vi "Result Database Logging Engine.vi"(11 "Sequence Context":T1) -> (0 "error out":errorcluster)   [LabVIEW 2023, in "HardwareAbstractionLayer_LVOOP.lvlib" / "Report.lvclass"]
uses:
  Report.lvclass
  Report.lvclass/Report.ctl
  Database/Database.lvclass
  Database/SQL Public VI/Control/DB Options.ctl
  Control/Q Data.ctl
  Control/UUT Test Info.ctl
  Control/FE FRAME LOG.ctl
  Control/LIMIT TABLE.ctl
  Control/ERROR LOG.ctl
  Teststand/Teststand.lvclass
  Control/FF FRAME LOG.ctl
  Control/FA FRAME LOG.ctl
  Control/ERROR LOG APPEND.ctl
  Control/TEST RESULT LOG.ctl
  Control/TEST RESULT LOG APPEND.ctl
  Control/SYSTEM LOG.ctl
  Control/Temperature LOG.ctl
  Control/POWER STATUS.ctl
  Control/CYCLE_DURATION_LOG.ctl
  Control/FE FF DECODER.ctl
  <vilib>/addons/TestStand/_TSUtility.llb/TestStand - Get Property Value (Boolean).vi
  Control/Queue FGV.ctl
  <vilib>/addons/TestStand/_TSLegacy.llb/LabVIEW Test - Sequence Context.ctl
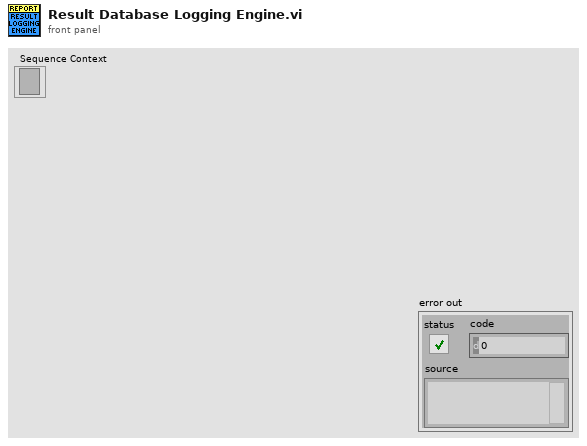
[diagram p1: front panel]
types:
  T1 = typedef "LabVIEW Test - Sequence Context.ctl" = refnum<k7>
  T2 = typedef "HardwareAbstractionLayer_LVOOP.lvlib/Report.lvclass/Queue FGV.ctl" = enum16{"Init", "Set", "Get"}
  T3 = typedef "HardwareAbstractionLayer_LVOOP.lvlib/Database.lvclass/DB Options.ctl" = enum16{"Init", "Select Data", "Insert Data", "Update Data", "Delete Data", "Execute Query", "Create Schema", "Create Table", "List Tables", "List Columns", "Close"}
  T4 = typedef "HardwareAbstractionLayer_LVOOP.lvlib/Report.lvclass/Q Data.ctl" = cluster{"Table Name":string, "Data":variant, "Action":enum16{"Insert", "Update"}, "Schema":string, "Socket No":u16}
  T5 = typedef "TestStand - Status Monitor.ctl" = cluster{"Sequence Context":refnum<k7>, "Execution":refnum<k7>, "Termination Monitor":refnum<k7>}
  T6 = typedef "HardwareAbstractionLayer_LVOOP.lvlib/Report.lvclass/UUT Test Info.ctl" = cluster{"ID":string, "STATION_ID":string, "TEST_SOCKET_INDEX":string, "UUT_SERIAL_NUMBER":string, "TSW_VER":string, "VAL_SW_VER":string, "PROJECT_NAME":string, "PRODUCT_NAME":string, "PRODUCT_VARIANT":string, "TEST_NAME":string, "TEST_PHASE":string, "TEST_DESCRIPTION":string, "TEMP_CHAMBER_NAME":string, "START_DATE_TIME":string, "STOP_DATE_TIME ":string, "START_CYCLE_COUNT":string, "STOP_CYCLE_COUNT":string, "EXECUTION_TIME":string, "UUT_STATUS":string, "UUT_ERROR_CODE":string, "UUT_ERROR_MESSAGE":string, "TEST_SEQUENCE":string}
  T7 = typedef "HardwareAbstractionLayer_LVOOP.lvlib/Report.lvclass/FE FF DECODER.ctl" = cluster{"UUT_TEST_INFO":string, "SOCKET_NUMBER":string, "Decoder_Frame_Type":string, "CYCLE_NUMBER":string, "TEST_MODE":string}
  T8 = typedef "HardwareAbstractionLayer_LVOOP.lvlib/Report.lvclass/FA FRAME LOG.ctl" = cluster{"UUT_TEST_INFO":string, "CAN_FRAME_RX":string, "CAN_FRAME_RX_NO_OFF_BYTE":string}
  T9 = typedef "HardwareAbstractionLayer_LVOOP.lvlib/Report.lvclass/FE FRAME LOG.ctl" = cluster{"ID":string, "UUT_TEST_INFO":string, "DATE_TIME":string, "CYCLE_NUMBER":string, "TEST_MODE":string, "CHAMBER_TEMP":string, "CAN_FRAME_RX":string, "Test Mode":u32, "LV_PPS_VOLTAGE":string, "LV_PPS_CURRENT":string, "HV_PPS_VOLTAGE":string, "HV_PPS_CURRENT":string, "SOCKET_NUMBER":string, "CAN_FRAME_RX_NO_OFF_BYTE":string}
  T10 = typedef "HardwareAbstractionLayer_LVOOP.lvlib/Report.lvclass/FF FRAME LOG.ctl" = cluster{"ID":string, "UUT_TEST_INFO":string, "DATE_TIME":string, "CYCLE_NUMBER":string, "TEST_MODE":string, "CAN_FRAME_RX":string, "CHAMBER_TEMP":string, "TestMode":u32, "SOCKET_NUMBER":string, "CAN_FRAME_RX_NO_OFF_BYTE":string}
  T11 = typedef "HardwareAbstractionLayer_LVOOP.lvlib/Report.lvclass/LIMIT TABLE.ctl" = cluster{"ID":string, "PRODUCT_NAME":string, "PRODUCT_VARIANT":string, "TEST_MODE":string, "PARAMETER_NAME":string, "COMPARISON_TYPE":string, "LOW_LIMIT":string, "HIGH_LIMIT":string, "UNIT":string, "ERROR_MESSSAGE":string, "SEVERITY":string}
  T12 = typedef "HardwareAbstractionLayer_LVOOP.lvlib/Report.lvclass/ERROR LOG APPEND.ctl" = T13[]
  T13 = typedef "HardwareAbstractionLayer_LVOOP.lvlib/Report.lvclass/ERROR LOG.ctl" = cluster{"ID":string, "UUT_TEST_INFO":string, "DATE_TIME":string, "CYCLE_NUMBER":string, "TEST_MODE":string, "SIGNAL_NAME":string, "SIGNAL_VALUE":string, "UNIT":string, "COMPARISON_VALUE":string, "ERROR_MESSAGE":string, "FRAME_TYPE":string, "LIMITID":string, "SOCKET_NUMBER":string}
  T14 = typedef "HardwareAbstractionLayer_LVOOP.lvlib/Report.lvclass/TEST RESULT LOG APPEND.ctl" = T15[]
  T15 = typedef "HardwareAbstractionLayer_LVOOP.lvlib/Report.lvclass/TEST RESULT LOG.ctl" = cluster{"ID":string, "UUT_TEST_INFO":string, "DATE_TIME":string, "CYCLE_NUMBER":string, "TEST_MODE":string, "SIGNAL_NAME":string, "SIGNAL_VALUE":string, "COMPARISON_VALUE":string, "ERROR_MESSAGE":string, "FRAME_TYPE":string, "LIMITID":string, "TEST_RESULT":string, "SOCKET_NUMBER":string}
  T16 = typedef "HardwareAbstractionLayer_LVOOP.lvlib/Report.lvclass/SYSTEM LOG.ctl" = cluster{"ID ":string, "DATE_TIME":string, "CYCLE_NUMBER":string, "TEST_MODE":string, "ERROR_MESSAGE":string}
  T17 = typedef "HardwareAbstractionLayer_LVOOP.lvlib/Report.lvclass/Temperature LOG.ctl" = cluster{"TEST_MODE":string, "CYCLE_NUMBER":string, "TEMPERATURE":cluster{"LV_PPS_TEMPERATURE":dbl, "HV_PPS1_TEMPERATURE":dbl, "HV_PPS2_TEMPERATURE":dbl, "HV_PPS3_TEMPERATURE":dbl, "HV_PPS4_TEMPERATURE":dbl, "HV_PPS5_TEMPERATURE":dbl, "HV_PPS6_TEMPERATURE":dbl, "CHAMBER_TEMPERATURE":dbl, "LOAD_U1_TEMPERATURE":dbl, "LOAD_V1_TEMPERATURE":dbl, "LOAD_W1_TEMPERATURE":dbl, "LOAD_U2_TEMPERATURE":dbl, "LOAD_V2_TEMPERATURE":dbl, "LOAD_W2_TEMPERATURE":dbl, "LOAD_U3_TEMPERATURE":dbl, "LOAD_V3_TEMPERATURE":dbl, "LOAD_W3_TEMPERATURE":dbl}, "Temperature Inrange":cluster{"LVPPS_Trip?":bool, "HVPPS1_Trip?":bool, "HVPPS2_Trip?":bool, "HVPPS3_Trip?":bool, "HVPPS4_Trip?":bool, "HVPPS5_Trip?":bool, "HVPPS6_Trip?":bool, "Chamber_Trip?":bool}}
  T18 = typedef "HardwareAbstractionLayer_LVOOP.lvlib/Report.lvclass/POWER STATUS.ctl" = cluster{"TEST_MODE":string, "CYCLE_NUMBER":string, "TYPE_POWER":string, "STATE":string}
  T19 = typedef "HardwareAbstractionLayer_LVOOP.lvlib/Report.lvclass/CYCLE_DURATION_LOG.ctl" = cluster{"CYCLE_NUMBER":string}
  T20 = typedef "HardwareAbstractionLayer_LVOOP.lvlib/Report.lvclass/Result FGV Data.ctl" = cluster{"Project Name":string, "Product Name":string, "Product Varient":string, "Test Name":string, "Test Phase":string, "Test Description":string, "Temp Chamber Name":string, "Schema":string, "Total No of Cycles":u32, "Current Cycle Number":u32, "Cycle Duration":u32, "Current Test Mode":string}
  T21 = cluster{"LV_PPS_TEMPERATURE":dbl, "HV_PPS1_TEMPERATURE":dbl, "HV_PPS2_TEMPERATURE":dbl, "HV_PPS3_TEMPERATURE":dbl, "HV_PPS4_TEMPERATURE":dbl, "HV_PPS5_TEMPERATURE":dbl, "HV_PPS6_TEMPERATURE":dbl, "CHAMBER_TEMPERATURE":dbl, "LOAD_U1_TEMPERATURE":dbl, "LOAD_V1_TEMPERATURE":dbl, "LOAD_W1_TEMPERATURE":dbl, "LOAD_U2_TEMPERATURE":dbl, "LOAD_V2_TEMPERATURE":dbl, "LOAD_W2_TEMPERATURE":dbl, "LOAD_U3_TEMPERATURE":dbl, "LOAD_V3_TEMPERATURE":dbl, "LOAD_W3_TEMPERATURE":dbl}
  T22 = cluster{"LVPPS_Trip?":bool, "HVPPS1_Trip?":bool, "HVPPS2_Trip?":bool, "HVPPS3_Trip?":bool, "HVPPS4_Trip?":bool, "HVPPS5_Trip?":bool, "HVPPS6_Trip?":bool, "Chamber_Trip?":bool}
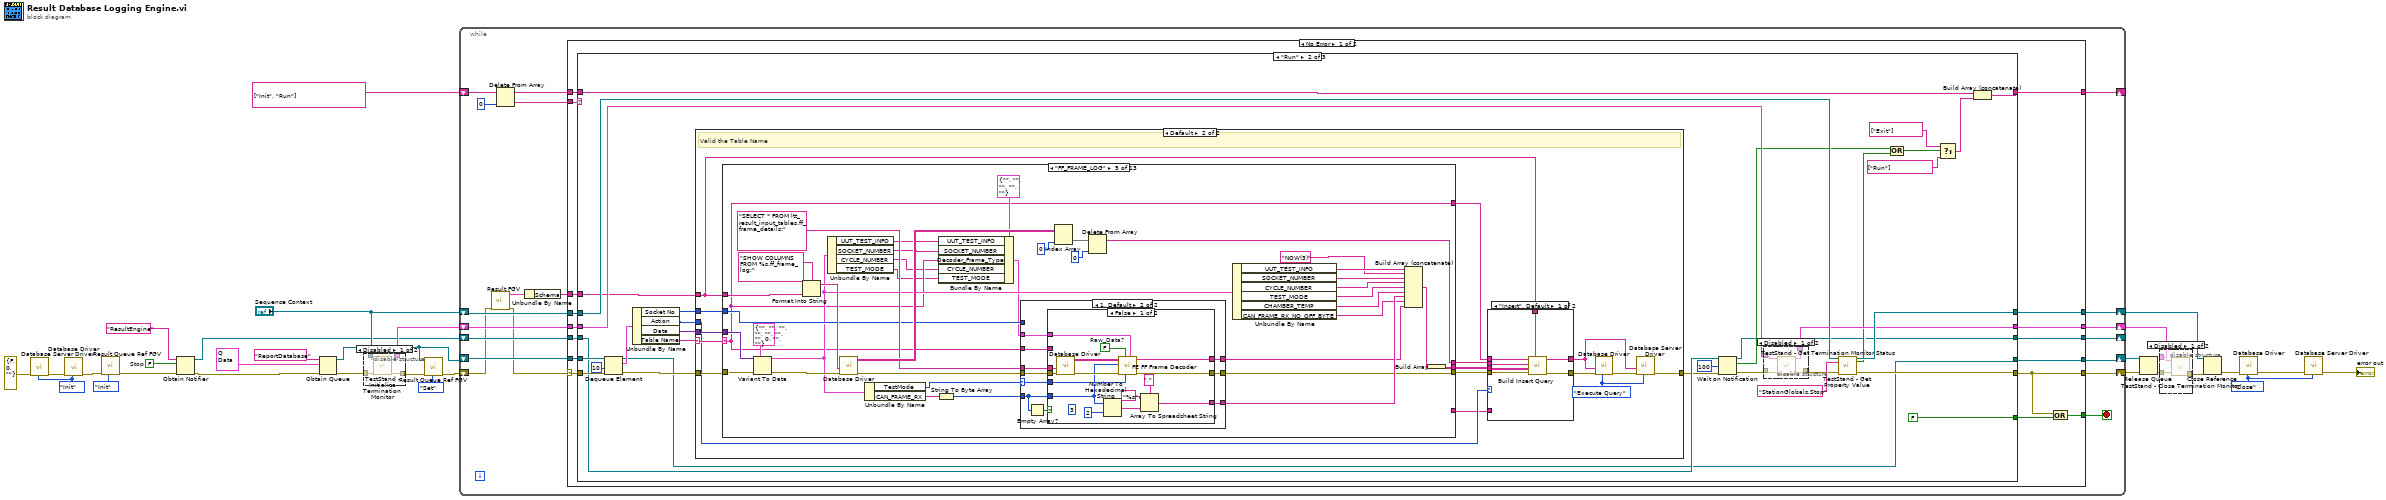
[diagram p0: block diagram]
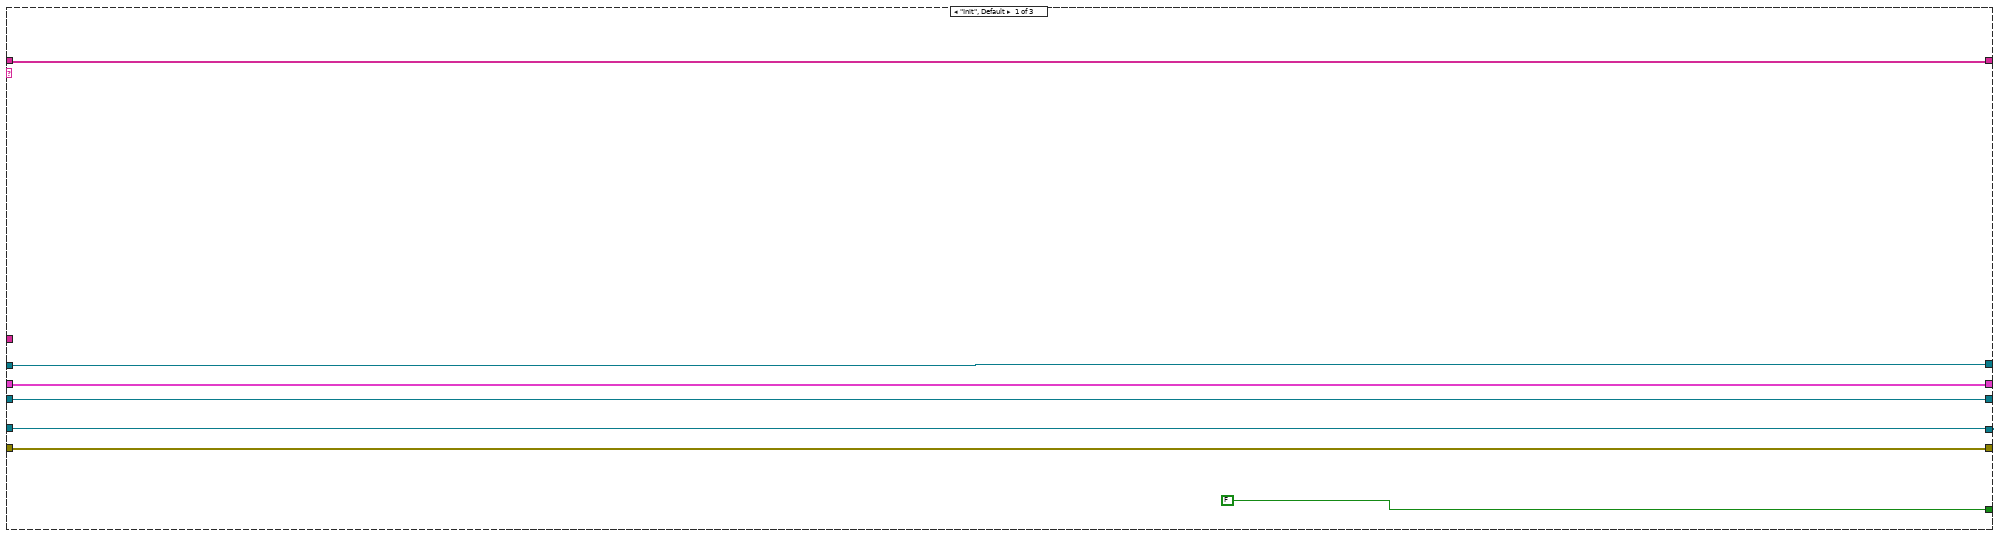
[diagram p4: hidden frame]
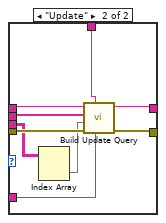
[diagram p7: hidden frame]
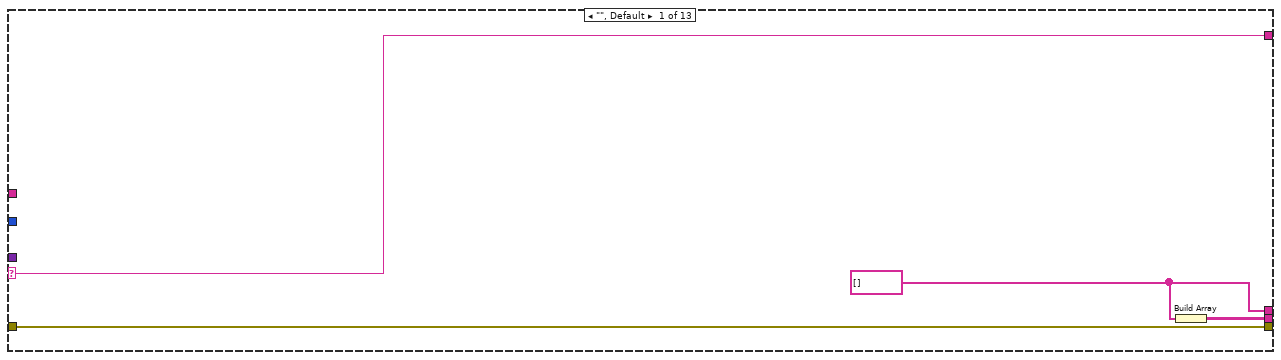
[diagram p8: hidden frame]
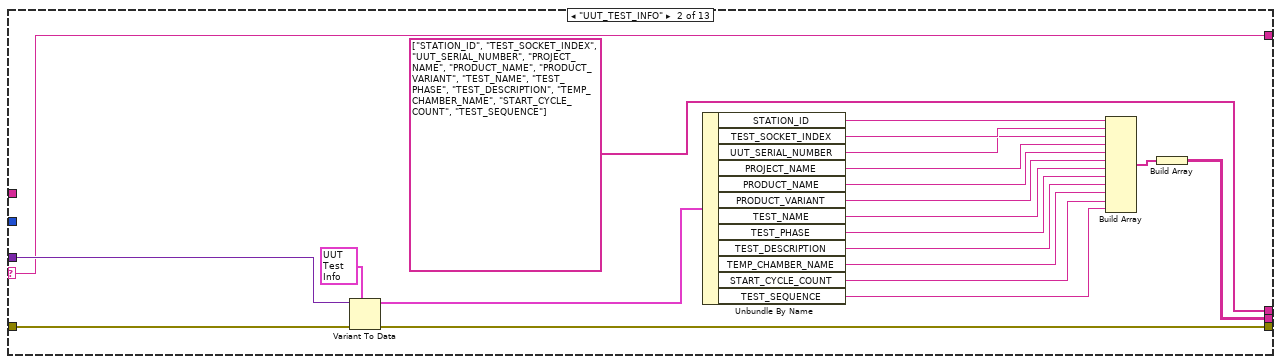
[diagram p9: hidden frame]
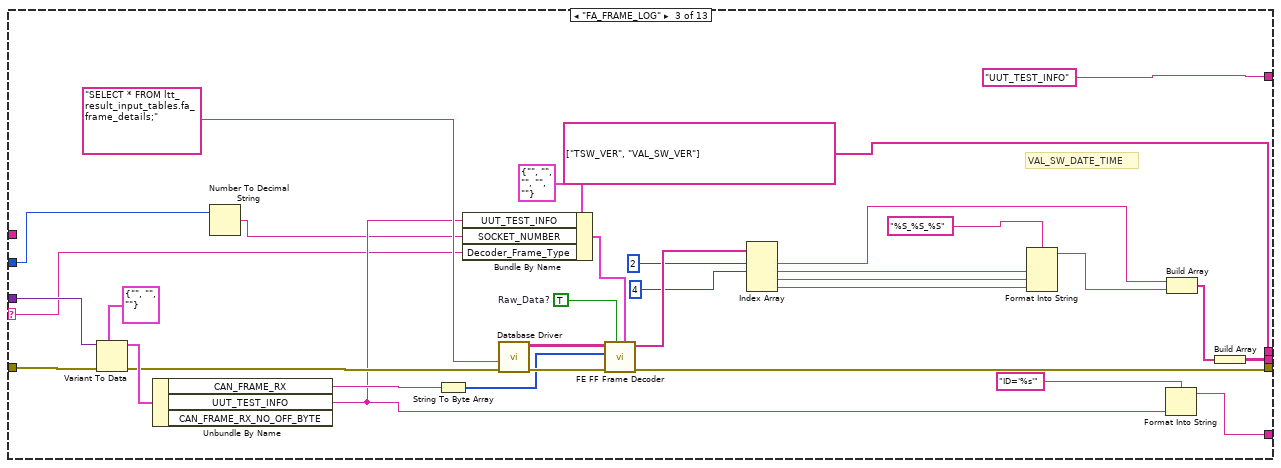
[diagram p10: hidden frame]
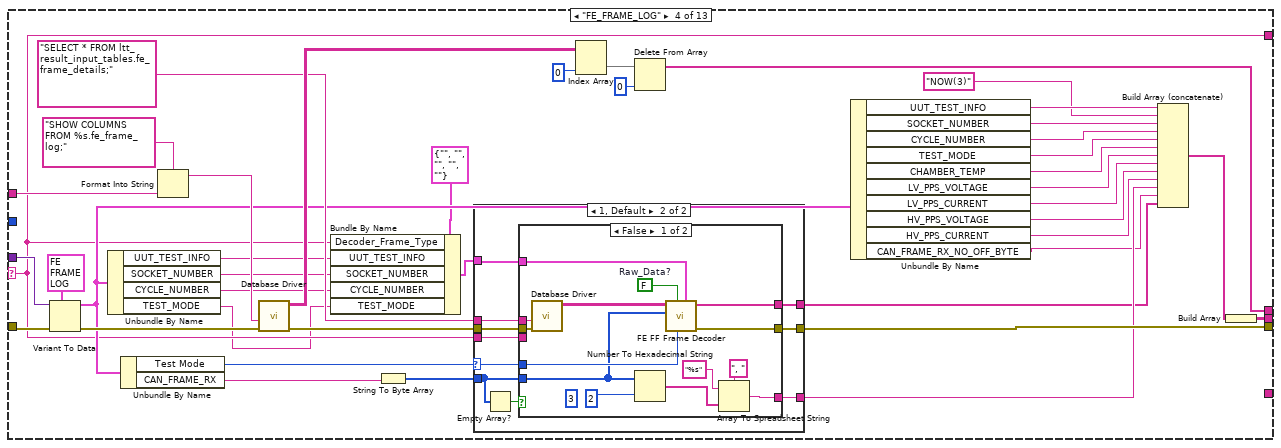
[diagram p11: hidden frame]
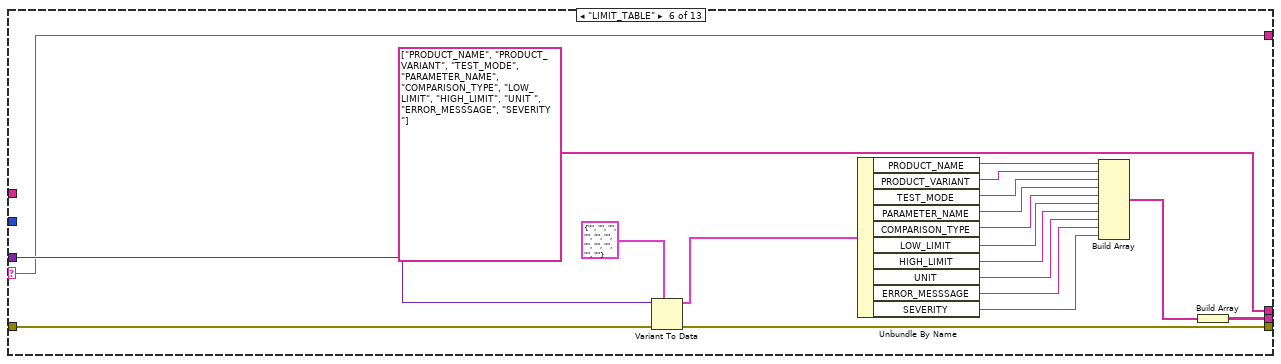
[diagram p16: hidden frame]
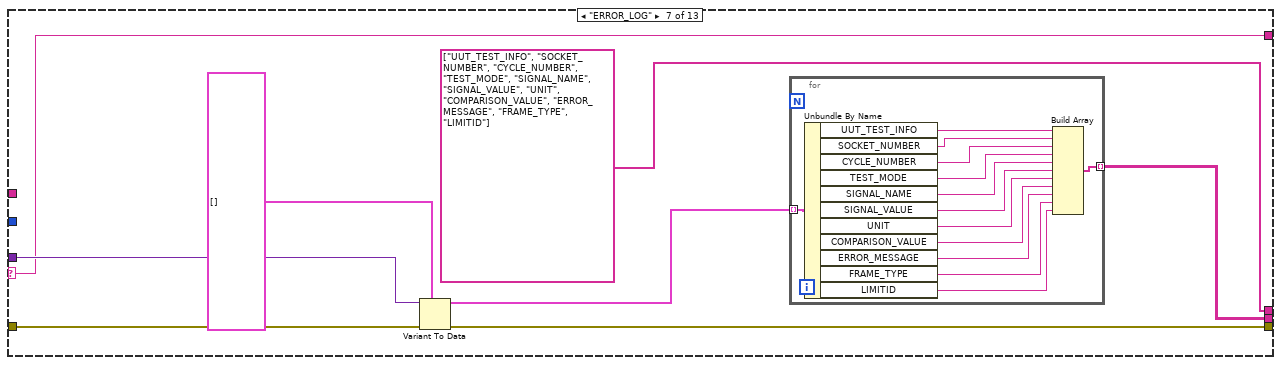
[diagram p17: hidden frame]
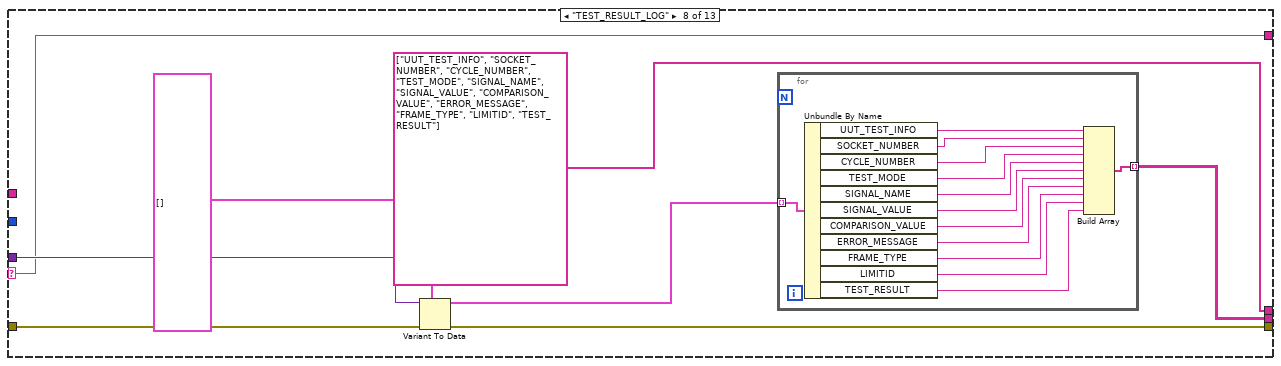
[diagram p18: hidden frame]
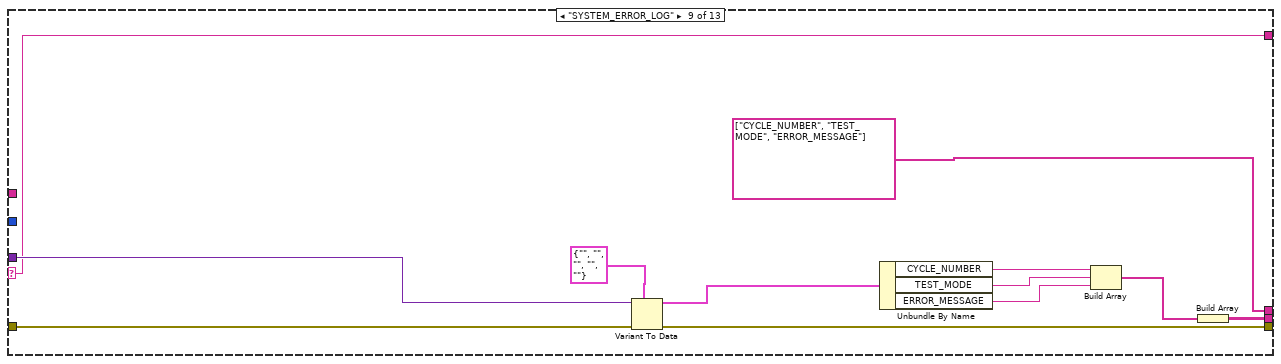
[diagram p19: hidden frame]
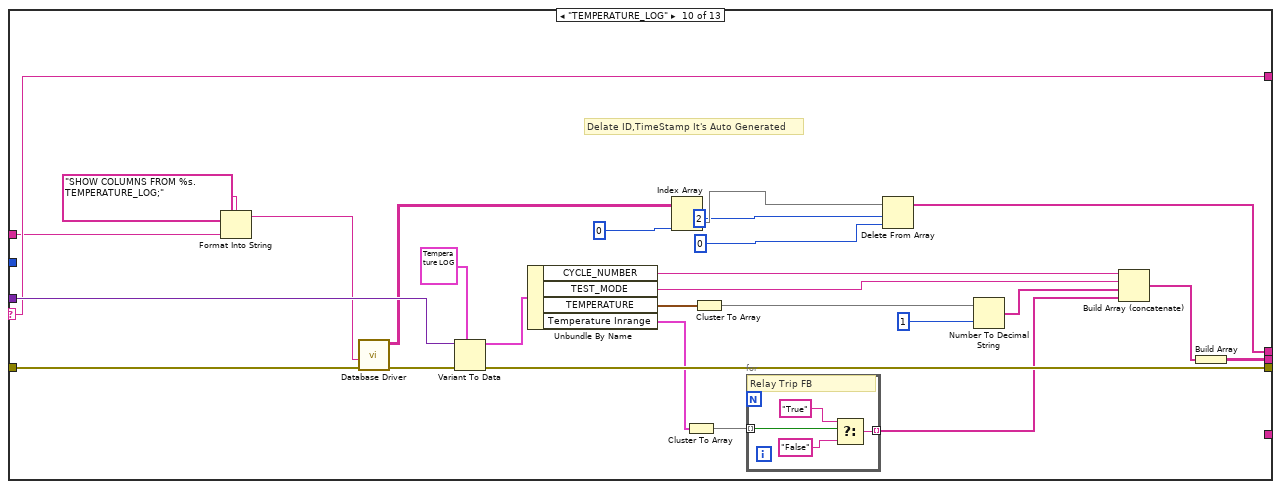
[diagram p20: hidden frame]
diagram:
  w8 = DB_Options."Close" ("Options")
  w11 = DB_Options."Init" ("Options")
  w18 = FALSE  # Stop
  n1 = call "Database Server Driver.vi"("Options"=w11, "error in"=errorcluster {"status"=FALSE, "code"=0, "source"=""}) -> ("error out"=w12:errorcluster)  [unwired: 6 in, 3 out]
  n2 = call "Database Driver.vi"("Options"=w11, "error in"=w12) -> ("error out"=w3:errorcluster)  [unwired: 6 in, 3 out]
  n3 = call "Result Queue Ref FGV.vi"("Q FGV"=Queue_FGV."Init", "error in"=w3) -> ("error out"=w2:errorcluster)  [unwired: 8 in, 1 out]
  n4 = Obtain Notifier(name (unnamed)="ResultEngine", notification data type=w18, error in (no error)=w2) -> (notifier out=w15:refnum<notifier>, error out=w16:errorcluster)  [unwired: 1 in, 1 out]
  n5 = Obtain Queue(name (unnamed)="ReportDatabase", element data type=T4 {"Table Name"="", "Data"=variant, "Action"=enum."Insert", "Schema"="", "Socket No"=1} ("Q Data"), error in (no error)=w16) -> (queue out=w7:refnum<queue>, error out=w26:errorcluster)  [unwired: 2 in, 1 out]
  n6 = disable-structure shown="Disabled" {
    disable-tunnel: "Sequence Context" -> [w34 _]
    disable-tunnel: w26 -> [w33 w35]
    disable-tunnel: [w32 _] -> w25
    disable-tunnel: [w31 w35] -> w6
    frame Disabled {
      n7 = call <vilib>:"TestStand - Initialize Termination Monitor.vi"("error in (no error)"=w33, "Sequence Context In"=w34) -> ("error out"=w31:errorcluster, "Status Monitor Out"=w32:T5)  [unwired: 8 in]
    }
    frame Enabled {
    }
  }
  n8 = call "Result Queue Ref FGV.vi"("Q FGV"=Queue_FGV."Set", "error in"=w6, "Set Queue"=w7) -> ("error out"=w5:errorcluster)  [unwired: 7 in, 1 out]
  n9 = while {
    shift-right: [w49] -> _
    shift-left: string[] ["Init", "Run"] -> [w53]
    shift-right: [w48] -> w22
    shift-left: w7 -> [w54]
    shift-right: [w46] -> w23
    shift-left: w5 -> [w37]
    shift-right: [w44] -> w19
    shift-left: "Sequence Context" -> [w45]
    shift-right: [w42] -> w24
    shift-left: w25 -> [w43]
    shift-right: [w40] -> _
    shift-left: w15 -> [w41]
    stop <- w47 stop-if-true
    n10 = call "Result FGV.vi"("error in"=w37) -> ("error out"=w36:errorcluster, "Result FGV Data Out"=w39:T20)  [unwired: 9 in]
    n11 = Delete From Array(array=w53, index=0) -> (deleted portion=w52:string, array with subset deleted=w50:string[])  [unwired: 1 in]
    n12 = Unbundle By Name(w39) -> ("Schema"=w38:string)
    n13 = case shown="No Error" w36 {
      selector: w36 -> [w69 w487]
      tunnel: w54 -> [w70 w486]
      tunnel: w52 -> [w68 _]
      tunnel: w50 -> [w67 _]
      tunnel: [w66 string[] []] -> w49
      tunnel: [w65 w486] -> w48
      tunnel: [w63 TRUE] -> w47
      tunnel: [w62 w487] -> w46
      tunnel: w45 -> [w61 w485]
      tunnel: [w60 w485] -> w44
      tunnel: w43 -> [w59 w484]
      tunnel: [w58 w484] -> w42
      tunnel: w41 -> [w57 w482]
      tunnel: [w56 w482] -> w40
      tunnel: w38 -> [w55 _]
      frame No Error {
        n14 = case shown="\"Run\"" w68 {
          tunnel: w70 -> [w77 w109 w480]
          tunnel: w69 -> [w76 w108 w479]
          tunnel: w67 -> [w75 w105 _]
          tunnel: [w77 w81 w480] -> w65
          tunnel: [w76 w98 w479] -> w62
          tunnel: [w75 w103 string[] ["Exit"]] -> w66
          tunnel: [FALSE FALSE TRUE] -> w64
          tunnel: w61 -> [w73 w97 w476]
          tunnel: [w73 w96 w476] -> w60
          tunnel: w59 -> [w72 w95 w477]
          tunnel: [w72 w93 w477] -> w58
          tunnel: w57 -> [w71 w87 w475]
          tunnel: [w71 w84 w475] -> w56
          tunnel: w55 -> [_ w82 _]
          frame "Init", Default {
          }
          frame "Run" {
            n15 = Dequeue Element(queue=w109, timeout in ms (-1)=10, error in (no error)=w108) -> (queue out=w81:refnum<queue>, element=w107:T4, error out=w106:errorcluster)  [unwired: 1 out]
            n16 = Unbundle By Name(w107) -> ("Socket No"=w78:u16, "Action"=w101:enum16{"Insert", "Update"}, "Data"=w102:variant, "Table Name"=w80:string)
            n17 = case shown="Default" w80 {
              selector: w80 -> [_ w127]
              tunnel: w106 -> [w115 w131]
              tunnel: [w115 w117] -> w79
              tunnel: w102 -> [_ w130]
              tunnel: w101 -> [_ w124]
              tunnel: w82 -> [_ w128]
              tunnel: w78 -> [_ w121]
              frame "" {
              }
              frame Default {
                w118 = DB_Options."Execute Query" ("Options")
                # "Valid the Table Name"
                n18 = case shown="\"FF_FRAME_LOG\"" w127 {
                  selector: w127 -> [w148 w153 w175 w208 w276 w338 w357 w379 w400 w435 w445 w457 w467]
                  tunnel: w131 -> [w151 w172 w199 w234 w300 w355 w364 w385 w409 w424 w453 w463 w473]
                  tunnel: [w151 w171 w197 w232 w282 w354 w363 w384 w408 w436 w452 w462 w472] -> w116
                  tunnel: w130 -> [_ w170 w205 w246 w310 w356 w362 w383 w410 w437 w454 w464 w474]
                  tunnel: [w149 w157 w181 w230 w297 w340 w359 w381 w402 w426 w447 w459 w469] -> w126
                  tunnel: [w150 string[] ["STATION_ID", "TEST_SOCKET_INDEX", "UUT_SERIAL_NUMBER", "PROJECT_NAME", "PRODUCT_NAME", "PRODUCT_VARIANT", "TEST_NAME", "TEST_PHASE", "TEST_DESCRIPTION", "TEMP_CHAMBER_NAME", "START_CYCLE_COUNT", "TEST_SEQUENCE"] ("DB Column Name") string[] ["TSW_VER", "VAL_SW_VER"] w229 w296 string[] ["PRODUCT_NAME", "PRODUCT_VARIANT", "TEST_MODE", "PARAMETER_NAME", "COMPARISON_TYPE", "LOW_LIMIT", "HIGH_LIMIT", "UNIT ", "ERROR_MESSSAGE", "SEVERITY "] string[] ["UUT_TEST_INFO", "SOCKET_NUMBER", "CYCLE_NUMBER", "TEST_MODE", "SIGNAL_NAME", "SIGNAL_VALUE", "UNIT", "COMPARISON_VALUE", "ERROR_MESSAGE", "FRAME_TYPE", "LIMITID"] string[] ["UUT_TEST_INFO", "SOCKET_NUMBER", "CYCLE_NUMBER", "TEST_MODE", "SIGNAL_NAME", "SIGNAL_VALUE", "COMPARISON_VALUE", "ERROR_MESSAGE", "FRAME_TYPE", "LIMITID", "TEST_RESULT"] string[] ["CYCLE_NUMBER", "TEST_MODE", "ERROR_MESSAGE"] w428 string[] ["CYCLE_NUMBER", "TEST_MODE", "TYPE_POWER", "STATE"] string[] ["CYCLE_NUMBER"] string[] ["CYCLE_NUMBER"]] -> w125
                  tunnel: w128 -> [_ _ _ w228 w295 _ _ _ _ w422 _ _ _]
                  tunnel: [w148 w153 "UUT_TEST_INFO" w208 w276 w338 w357 w379 w400 w435 w445 w457 w467] -> w123
                  tunnel: [_ _ w179 _ _ _ _ _ _ _ _ _ _] -> w122
                  tunnel: w121 -> [_ _ w174 _ w287 _ _ _ _ _ _ _ _]
                  frame "", Default {
                    w150 = string[] [] ("data")
                    n19 = Build Array(w150) -> (w149:string[][])
                  }
                  frame "UUT_TEST_INFO" {
                    n20 = Variant To Data(error in=w172, type=T6 {"ID"="", "STATION_ID"="", "TEST_SOCKET_INDEX"="", "UUT_SERIAL_NUMBER"="", "TSW_VER"="", "VAL_SW_VER"="", "PROJECT_NAME"="", "PRODUCT_NAME"="", "PRODUCT_VARIANT"="", "TEST_NAME"="", "TEST_PHASE"="", "TEST_DESCRIPTION"="", "TEMP_CHAMBER_NAME"="", "START_DATE_TIME"="", "STOP_DATE_TIME "="", "START_CYCLE_COUNT"="", "STOP_CYCLE_COUNT"="", "EXECUTION_TIME"="", "UUT_STATUS"="", "UUT_ERROR_CODE"="", "UUT_ERROR_MESSAGE"="", "TEST_SEQUENCE"=""} ("UUT_TEST_INFO"), Variant=w170) -> (data=w155:T6, error out=w171:errorcluster)
                    n21 = Unbundle By Name(w155) -> ("STATION_ID"=w168:string, "TEST_SOCKET_INDEX"=w167:string, "UUT_SERIAL_NUMBER"=w166:string, "PROJECT_NAME"=w165:string, "PRODUCT_NAME"=w163:string, "PRODUCT_VARIANT"=w162:string, "TEST_NAME"=w164:string, "TEST_PHASE"=w161:string, "TEST_DESCRIPTION"=w160:string, "TEMP_CHAMBER_NAME"=w159:string, "START_CYCLE_COUNT"=w154:string, "TEST_SEQUENCE"=w152:string)
                    n22 = Build Array(w168, w167, w166, w165, w163, w162, w164, w161, w160, w159, w154, w152) -> (w158:string[])
                    n23 = Build Array(w158) -> (w157:string[][])
                  }
                  frame "FA_FRAME_LOG" {
                    w195 = TRUE  # Raw_Data?
                    # "VAL_SW_DATE_TIME"
                    n24 = Variant To Data(error in=w199, type=T8 {"UUT_TEST_INFO"="", "CAN_FRAME_RX"="", "CAN_FRAME_RX_NO_OFF_BYTE"=""} ("FA_FRAME_LOG"), Variant=w205) -> (data=w201:T8, error out=w198:errorcluster)
                    n25 = Unbundle By Name(w201) -> ("CAN_FRAME_RX"=w200:string, "UUT_TEST_INFO"=w177:string)  [unwired: 1 out]
                    n26 = Number To Decimal String(number=w174) -> (decimal integer string=w173:string)  [unwired: 1 in]
                    n27 = String To Byte Array(string=w200) -> (unsigned byte array=w196:u8[])
                    n28 = Bundle By Name(cluster=T7 {"UUT_TEST_INFO"="", "SOCKET_NUMBER"="", "Decoder_Frame_Type"="", "CYCLE_NUMBER"="", "TEST_MODE"=""} ("INFO"), "UUT_TEST_INFO"=w177, "SOCKET_NUMBER"=w173, "Decoder_Frame_Type"=w175) -> (w176:T7)
                    n29 = call "Database Driver.vi"("error in"=w198, "SQL query"="SELECT * FROM ltt_result_input_tables.fa_frame_details;") -> ("error out"=w203:errorcluster, "data"=w202:string[][])  [unwired: 6 in, 2 out]
                    n30 = call "FE FF Frame Decoder.vi"("INFO"=w176, "Raw_Data?"=w195, "error in (no error)"=w203, "Frame Data"=w196, "Frame Detail"=w202) -> ("error out"=w197:errorcluster, "Frame Detail With Value"=w191:string[])  [unwired: 4 in, 1 out]
                    n31 = Index Array(array=w191, index #1=2 ("index"), index #2=4 ("index")) -> (element #1=w183:string, element #2=w185:string, element #3=w186:string, element #4=w187:string)  [unwired: 2 in]
                    n32 = Format Into String(format string="%S_%S_%S", w185, w186, w187) -> (resulting string=w184:string)  [unwired: 2 in, 1 out]
                    n33 = Format Into String(format string="ID='%s'", w177) -> (resulting string=w179:string)  [unwired: 2 in, 1 out]
                    n34 = Build Array(w183, w184) -> (w182:string[])
                    n35 = Build Array(w182) -> (w181:string[][])
                  }
                  frame "FE_FRAME_LOG" {
                    n36 = Variant To Data(error in=w234, type=T9 {"ID"="", "UUT_TEST_INFO"="", "DATE_TIME"="", "CYCLE_NUMBER"="", "TEST_MODE"="", "CHAMBER_TEMP"="", "CAN_FRAME_RX"="", "Test Mode"=0, "LV_PPS_VOLTAGE"="", "LV_PPS_CURRENT"="", "HV_PPS_VOLTAGE"="", "HV_PPS_CURRENT"="", "SOCKET_NUMBER"="", "CAN_FRAME_RX_NO_OFF_BYTE"=""} ("FE_FRAME_LOG"), Variant=w246) -> (data=w222:T9, error out=w233:errorcluster)
                    n37 = Unbundle By Name(w222) -> ("UUT_TEST_INFO"=w211:string, "SOCKET_NUMBER"=w210:string, "CYCLE_NUMBER"=w207:string, "TEST_MODE"=w206:string)
                    n38 = Unbundle By Name(w222) -> ("Test Mode"=w223:u32, "CAN_FRAME_RX"=w235:string)
                    n39 = Format Into String(format string="SHOW COLUMNS FROM %s.fe_frame_log;" ("SQL query"), w228) -> (resulting string=w242:string)  [unwired: 2 in, 1 out]
                    n40 = call "Database Driver.vi"("error in"=w233, "SQL query"=w242) -> ("error out"=w237:errorcluster, "data"=w241:string[][])  [unwired: 6 in, 2 out]
                    n41 = Bundle By Name(cluster=T7 {"UUT_TEST_INFO"="", "SOCKET_NUMBER"="", "Decoder_Frame_Type"="", "CYCLE_NUMBER"="", "TEST_MODE"=""} ("INFO"), "Decoder_Frame_Type"=w208, "UUT_TEST_INFO"=w211, "SOCKET_NUMBER"=w210, "CYCLE_NUMBER"=w207, "TEST_MODE"=w206) -> (w209:T7)
                    n42 = String To Byte Array(string=w235) -> (unsigned byte array=w216:u8[])
                    n43 = case shown="1, Default" w223 {
                      selector: w223 -> [_ w252]
                      tunnel: w237 -> [w247 w257]
                      tunnel: "SELECT * FROM ltt_result_input_tables.fe_frame_details;" ("SQL query") -> [_ w256]
                      tunnel: [w247 w255] -> w232
                      tunnel: [_ w254] -> w214
                      tunnel: w208 -> [_ w253]
                      tunnel: w216 -> [_ w250]
                      tunnel: [_ w251] -> w215
                      tunnel: w209 -> [_ w248]
                      frame 0 {
                      }
                      frame 1, Default {
                        n44 = Empty Array?(array=w250) -> (empty?=w249:bool)
                        n45 = case shown="False" w249 {
                          tunnel: w257 -> [w271 w272]
                          tunnel: w256 -> [w270 _]
                          tunnel: [w268 w272] -> w255
                          tunnel: [w267 _] -> w254
                          tunnel: w253 -> [_ _]
                          tunnel: w252 -> [w265 _]
                          tunnel: w250 -> [w263 _]
                          tunnel: [w260 _] -> w251
                          tunnel: w248 -> [w258 _]
                          frame False {
                            (unwired) i16 3 ("width (-)")
                            w266 = FALSE  # Raw_Data?
                            n46 = call "Database Driver.vi"("error in"=w271, "SQL query"=w270) -> ("data"=w269:string[][])  [unwired: 6 in, 3 out]
                            n47 = Number To Hexadecimal String(1:i16 2 ("width (-)"), 2:w263) -> (0:w259:string[])
                            n48 = call "FE FF Frame Decoder.vi"("INFO"=w258, "Test Mode"=w265, "Raw_Data?"=w266, "Frame Data"=w263, "Frame Detail"=w269) -> ("error out"=w268:errorcluster, "Frame Detail With Value"=w267:string[])  [unwired: 4 in, 1 out]
                            n49 = Array To Spreadsheet String(delimiter (Tab)=", ", array=w259, 3:"%s" ("format string")) -> (spreadsheet string=w260:string)
                          }
                          frame True {
                            # "Emety Data"
                          }
                        }
                      }
                    }
                    n50 = Index Array(array=w241, index (col)=0 ("disabled index (col)")) -> (element=w239:string[])  [unwired: 1 in]
                    n51 = Delete From Array(array=w239, index=0) -> (array with subset deleted=w229:string[])  [unwired: 1 in, 1 out]
                    n52 = Unbundle By Name(w222) -> ("UUT_TEST_INFO"=w244:string, "SOCKET_NUMBER"=w217:string, "CYCLE_NUMBER"=w224:string, "TEST_MODE"=w225:string, "CHAMBER_TEMP"=w226:string, "LV_PPS_VOLTAGE"=w221:string, "LV_PPS_CURRENT"=w220:string, "HV_PPS_VOLTAGE"=w219:string, "HV_PPS_CURRENT"=w218:string, "CAN_FRAME_RX_NO_OFF_BYTE"=w213:string)
                    n53 = Build Array (concatenate)(w244, "NOW(3)" ("element"), w217, w224, w225, w226, w221, w220, w219, w218, w215, w213, w214) -> (w231:string[])
                    n54 = Build Array(w231) -> (w230:string[][])
                  }
                  frame "FF_FRAME_LOG" {
                    n55 = Variant To Data(error in=w300, type=T10 {"ID"="", "UUT_TEST_INFO"="", "DATE_TIME"="", "CYCLE_NUMBER"="", "TEST_MODE"="", "CAN_FRAME_RX"="", "CHAMBER_TEMP"="", "TestMode"=0, "SOCKET_NUMBER"="", "CAN_FRAME_RX_NO_OFF_BYTE"=""} ("FF_FRAME_LOG"), Variant=w310) -> (data=w286:T10, error out=w299:errorcluster)
                    n56 = Format Into String(format string="SHOW COLUMNS FROM %s.ff_frame_log;" ("SQL query"), w295) -> (resulting string=w307:string)  [unwired: 2 in, 1 out]
                    n57 = Unbundle By Name(w286) -> ("UUT_TEST_INFO"=w277:string, "SOCKET_NUMBER"=w278:string, "CYCLE_NUMBER"=w274:string, "TEST_MODE"=w273:string)
                    n58 = call "Database Driver.vi"("error in"=w299, "SQL query"=w307) -> ("error out"=w289:errorcluster, "data"=w306:string[][])  [unwired: 6 in, 2 out]
                    n59 = Unbundle By Name(w286) -> ("TestMode"=w288:u32, "CAN_FRAME_RX"=w301:string)
                    n60 = String To Byte Array(string=w301) -> (unsigned byte array=w284:u8[])
                    n61 = Bundle By Name(cluster=T7 {"UUT_TEST_INFO"="", "SOCKET_NUMBER"="", "Decoder_Frame_Type"="", "CYCLE_NUMBER"="", "TEST_MODE"=""} ("INFO"), "UUT_TEST_INFO"=w277, "SOCKET_NUMBER"=w278, "Decoder_Frame_Type"=w276, "CYCLE_NUMBER"=w274, "TEST_MODE"=w273) -> (w275:T7)
                    n62 = case shown="1, Default" w288 {
                      selector: w288 -> [_ w317]
                      tunnel: "SELECT * FROM ltt_result_input_tables.ff_frame_details;" ("SQL query") -> [_ w321]
                      tunnel: [w311 w320] -> w282
                      tunnel: w289 -> [w311 w319]
                      tunnel: [_ w318] -> w281
                      tunnel: w276 -> [_ w316]
                      tunnel: w287 -> [_ _]
                      tunnel: w284 -> [_ w314]
                      tunnel: [_ w315] -> w283
                      tunnel: w275 -> [_ w312]
                      frame 0 {
                      }
                      frame 1, Default {
                        n63 = Empty Array?(array=w314) -> (empty?=w313:bool)
                        n64 = case shown="False" w313 {
                          tunnel: w321 -> [w336 _]
                          tunnel: [w335 w337] -> w320
                          tunnel: w319 -> [w334 w337]
                          tunnel: [w333 _] -> w318
                          tunnel: w317 -> [w329 _]
                          tunnel: w316 -> [_ _]
                          tunnel: [w324 _] -> w315
                          tunnel: w314 -> [w323 _]
                          tunnel: w312 -> [w322 _]
                          frame False {
                            (unwired) i16 3 ("width (-)")
                            w330 = FALSE  # Raw_Data?
                            n65 = call "Database Driver.vi"("error in"=w334, "SQL query"=w336) -> ("error out"=w332:errorcluster, "data"=w331:string[][])  [unwired: 6 in, 2 out]
                            n66 = Number To Hexadecimal String(1:i16 2 ("width (-)"), 2:w323) -> (0:w325:string[])
                            n67 = call "FE FF Frame Decoder.vi"("INFO"=w322, "Test Mode"=w329, "Raw_Data?"=w330, "error in (no error)"=w332, "Frame Data"=w323, "Frame Detail"=w331) -> ("error out"=w335:errorcluster, "Frame Detail With Value"=w333:string[])  [unwired: 3 in, 1 out]
                            n68 = Array To Spreadsheet String(delimiter (Tab)=",", array=w325, 3:"%s" ("format string")) -> (spreadsheet string=w324:string)
                          }
                          frame True {
                            # "Emety Data"
                          }
                        }
                      }
                    }
                    n69 = Index Array(array=w306, index (col)=0 ("disabled index (col)")) -> (element=w304:string[])  [unwired: 1 in]
                    n70 = Delete From Array(array=w304, index=0) -> (array with subset deleted=w296:string[])  [unwired: 1 in, 1 out]
                    n71 = Unbundle By Name(w286) -> ("UUT_TEST_INFO"=w309:string, "SOCKET_NUMBER"=w285:string, "CYCLE_NUMBER"=w291:string, "TEST_MODE"=w292:string, "CHAMBER_TEMP"=w293:string, "CAN_FRAME_RX_NO_OFF_BYTE"=w280:string)
                    n72 = Build Array (concatenate)(w309, "NOW(3)" ("element"), w285, w291, w292, w293, w283, w280, w281) -> (w298:string[])
                    n73 = Build Array(w298) -> (w297:string[][])
                  }
                  frame "LIMIT_TABLE" {
                    n74 = Variant To Data(error in=w355, type=T11 {"ID"="", "PRODUCT_NAME"="", "PRODUCT_VARIANT"="", "TEST_MODE"="", "PARAMETER_NAME"="", "COMPARISON_TYPE"="", "LOW_LIMIT"="", "HIGH_LIMIT"="", "UNIT"="", "ERROR_MESSSAGE"="", "SEVERITY"=""} ("LIMIT_TABLE"), Variant=w356) -> (data=w352:T11, error out=w354:errorcluster)
                    n75 = Unbundle By Name(w352) -> ("PRODUCT_NAME"=w351:string, "PRODUCT_VARIANT"=w350:string, "TEST_MODE"=w349:string, "PARAMETER_NAME"=w348:string, "COMPARISON_TYPE"=w347:string, "LOW_LIMIT"=w346:string, "HIGH_LIMIT"=w345:string, "UNIT"=w344:string, "ERROR_MESSSAGE"=w343:string, "SEVERITY"=w342:string)
                    n76 = Build Array(w351, w350, w349, w348, w347, w346, w345, w344, w343, w342) -> (w341:string[])
                    n77 = Build Array(w341) -> (w340:string[][])
                  }
                  frame "ERROR_LOG" {
                    n78 = Variant To Data(error in=w364, type=T12 [] ("ERROR LOG Append"), Variant=w362) -> (data=w360:T12, error out=w363:errorcluster)
                    n79 = for {
                      tunnel: w360 -> [w377] mode=indexing
                      tunnel: [w371] -> w359 mode=indexing
                      n80 = Unbundle By Name(w377) -> ("UUT_TEST_INFO"=w376:string, "SOCKET_NUMBER"=w366:string, "CYCLE_NUMBER"=w375:string, "TEST_MODE"=w374:string, "SIGNAL_NAME"=w373:string, "SIGNAL_VALUE"=w372:string, "UNIT"=w365:string, "COMPARISON_VALUE"=w370:string, "ERROR_MESSAGE"=w369:string, "FRAME_TYPE"=w368:string, "LIMITID"=w367:string)
                      n81 = Build Array(w376, w366, w375, w374, w373, w372, w365, w370, w369, w368, w367) -> (w371:string[])
                    }
                  }
                  frame "TEST_RESULT_LOG" {
                    n82 = Variant To Data(error in=w385, type=T14 [] ("TEST RESULT LOG Append"), Variant=w383) -> (data=w382:T14, error out=w384:errorcluster)
                    n83 = for {
                      tunnel: w382 -> [w398] mode=indexing
                      tunnel: [w392] -> w381 mode=indexing
                      n84 = Unbundle By Name(w398) -> ("UUT_TEST_INFO"=w397:string, "SOCKET_NUMBER"=w386:string, "CYCLE_NUMBER"=w396:string, "TEST_MODE"=w395:string, "SIGNAL_NAME"=w394:string, "SIGNAL_VALUE"=w393:string, "COMPARISON_VALUE"=w391:string, "ERROR_MESSAGE"=w390:string, "FRAME_TYPE"=w389:string, "LIMITID"=w388:string, "TEST_RESULT"=w387:string)
                      n85 = Build Array(w397, w386, w396, w395, w394, w393, w391, w390, w389, w388, w387) -> (w392:string[])
                    }
                  }
                  frame "SYSTEM_ERROR_LOG" {
                    n86 = Variant To Data(error in=w409, type=T16 {"ID "="", "DATE_TIME"="", "CYCLE_NUMBER"="", "TEST_MODE"="", "ERROR_MESSAGE"=""} ("SYSTEM_LOG"), Variant=w410) -> (data=w407:T16, error out=w408:errorcluster)
                    n87 = Unbundle By Name(w407) -> ("CYCLE_NUMBER"=w406:string, "TEST_MODE"=w405:string, "ERROR_MESSAGE"=w404:string)
                    n88 = Build Array(w406, w405, w404) -> (w403:string[])
                    n89 = Build Array(w403) -> (w402:string[][])
                  }
                  frame "TEMPERATURE_LOG" {
                    # "Delate ID,TimeStamp It's Auto Generated"
                    n90 = Format Into String(format string="SHOW COLUMNS FROM %s.TEMPERATURE_LOG;" ("SQL query"), w422) -> (resulting string=w420:string)  [unwired: 2 in, 1 out]
                    n91 = call "Database Driver.vi"("error in"=w424, "SQL query"=w420) -> ("error out"=w423:errorcluster, "data"=w433:string[][])  [unwired: 6 in, 2 out]
                    n92 = Variant To Data(error in=w423, type=T17 {"TEST_MODE"="", "CYCLE_NUMBER"="", "TEMPERATURE"={"LV_PPS_TEMPERATURE"=0.0, "HV_PPS1_TEMPERATURE"=0.0, "HV_PPS2_TEMPERATURE"=0.0, "HV_PPS3_TEMPERATURE"=0.0, "HV_PPS4_TEMPERATURE"=0.0, "HV_PPS5_TEMPERATURE"=0.0, "HV_PPS6_TEMPERATURE"=0.0, "CHAMBER_TEMPERATURE"=0.0, "LOAD_U1_TEMPERATURE"=0.0, "LOAD_V1_TEMPERATURE"=0.0, "LOAD_W1_TEMPERATURE"=0.0, "LOAD_U2_TEMPERATURE"=0.0, "LOAD_V2_TEMPERATURE"=0.0, "LOAD_W2_TEMPERATURE"=0.0, "LOAD_U3_TEMPERATURE"=0.0, "LOAD_V3_TEMPERATURE"=0.0, "LOAD_W3_TEMPERATURE"=0.0}, "Temperature Inrange"={"LVPPS_Trip?"=FALSE, "HVPPS1_Trip?"=FALSE, "HVPPS2_Trip?"=FALSE, "HVPPS3_Trip?"=FALSE, "HVPPS4_Trip?"=FALSE, "HVPPS5_Trip?"=FALSE, "HVPPS6_Trip?"=FALSE, "Chamber_Trip?"=FALSE}} ("Temperature log"), Variant=w437) -> (data=w419:T17, error out=w436:errorcluster)
                    n93 = Unbundle By Name(w419) -> ("CYCLE_NUMBER"=w416:string, "TEST_MODE"=w417:string, "TEMPERATURE"=w418:T21, "Temperature Inrange"=w413:T22)
                    n94 = Index Array(array=w433, index (col)=0 ("disabled index (col)")) -> (element=w432:string[])  [unwired: 1 in]
                    n95 = Cluster To Array(cluster=w413) -> (array=w412:bool[])
                    n96 = Cluster To Array(cluster=w418) -> (array=w427:dbl[])
                    n97 = for {
                      tunnel: w412 -> [w441] mode=indexing
                      tunnel: [w440] -> w411 mode=indexing
                      # "Relay Trip FB"
                      n98 = Select(t="True", s=w441, f="False") -> (s? t:f=w440:string)
                    }
                    n99 = Delete From Array(array=w432, length=2, index=0) -> (array with subset deleted=w428:string[])  [unwired: 1 out]
                    n100 = Number To Decimal String(number=w427, width (-)=i16 1) -> (decimal integer string=w415:string[])
                    n101 = Build Array (concatenate)(w416, w417, w415, w411) -> (w414:string[])
                    n102 = Build Array(w414) -> (w426:string[][])
                  }
                  frame "POWER_STATUS_LOG" {
                    n103 = Variant To Data(error in=w453, type=T18 {"TEST_MODE"="", "CYCLE_NUMBER"="", "TYPE_POWER"="", "STATE"=""} ("POWER_STATUS"), Variant=w454) -> (data=w451:T18, error out=w452:errorcluster)
                    n104 = Unbundle By Name(w451) -> ("CYCLE_NUMBER"=w442:string, "TEST_MODE"=w443:string, "TYPE_POWER"=w450:string, "STATE"=w449:string)
                    n105 = Build Array(w442, w443, w450, w449) -> (w448:string[])
                    n106 = Build Array(w448) -> (w447:string[][])
                  }
                  frame "CYCLE_OFF_DURATION_LOG" {
                    n107 = Variant To Data(error in=w463, type=T19 {"CYCLE_NUMBER"=""} ("CYCLE_DURATION_LOG"), Variant=w464) -> (data=w461:T19, error out=w462:errorcluster)
                    n108 = Unbundle By Name(w461) -> ("CYCLE_NUMBER"=w456:string)
                    n109 = Build Array(w456) -> (w460:string[])
                    n110 = Build Array(w460) -> (w459:string[][])
                  }
                  frame "CYCLE_ON_DURATION_LOG" {
                    n111 = Variant To Data(error in=w473, type=T19 {"CYCLE_NUMBER"=""} ("CYCLE_DURATION_LOG"), Variant=w474) -> (data=w471:T19, error out=w472:errorcluster)
                    n112 = Unbundle By Name(w471) -> ("CYCLE_NUMBER"=w466:string)
                    n113 = Build Array(w466) -> (w470:string[])
                    n114 = Build Array(w470) -> (w469:string[][])
                  }
                }
                n115 = case shown="\"Insert\", Default" w124 {
                  tunnel: [w138 w146] -> w129
                  tunnel: [w137 w140] -> w119
                  tunnel: w128 -> [w136 w145]
                  tunnel: w123 -> [w135 w144]
                  tunnel: w116 -> [w134 w147]
                  tunnel: w126 -> [w133 w142]
                  tunnel: w125 -> [w132 w143]
                  tunnel: w122 -> [_ w139]
                  frame "Insert", Default {
                    n116 = call "Build Insert Query.vi"("Schema Name"=w136, "error in (no error)"=w134, "Data"=w133, "Column Names"=w132, "Table Name"=w135) -> ("error out"=w138:errorcluster, "SQL"=w137:string)  [unwired: 5 in]
                  }
                  frame "Update" {
                    n117 = Index Array(array=w142) -> (element=w141:string[])  [unwired: 2 in]
                    n118 = call "Build Update Query.vi"("Where"=w139, "Schema Name"=w145, "error in (no error)"=w147, "Data"=w141, "Column Names"=w143, "Table Name"=w144) -> ("error out"=w146:errorcluster, "SQL"=w140:string)  [unwired: 4 in]
                  }
                }
                n119 = call "Database Driver.vi"("Options"=w118, "error in"=w129, "SQL query"=w119) -> ("error out"=w120:errorcluster)  [unwired: 5 in, 3 out]
                n120 = call "Database Server Driver.vi"("Options"=w118, "error in"=w120, "SQL query"=w119) -> ("error out"=w117:errorcluster)  [unwired: 5 in, 3 out]
              }
            }
            n121 = Wait on Notification(notifier=w87, timeout in ms (-1)=100, error in (no error)=w79) -> (notifier out=w84:refnum<notifier>, notification=w85:bool, error out=w88:errorcluster)  [unwired: 1 in, 1 out]
            n122 = disable-structure shown="Disabled" {
              disable-tunnel: w95 -> [w113 _]
              disable-tunnel: [w112 w114] -> w94
              disable-tunnel: [w111 _] -> w93
              disable-tunnel: w88 -> [w110 w114]
              frame Disabled {
                n123 = call <vilib>:"TestStand - Get Termination Monitor Status.vi"("error in (no error)"=w110, "Status Monitor In"=w113) -> ("error out"=w112:errorcluster, "Status Monitor Out"=w111:T5)  [unwired: 7 in, 1 out]
              }
              frame Enabled {
              }
            }
            n124 = call-poly <vilib>:"TestStand - Get Property Value.vi"("Sequence Context In"=w97, "Lookup String"="StationGlobals.Stop", "error in (no error)"=w94) -> ("Sequence Context Out"=w96:refnum<k7>, "Value"=w89:bool, "error out"=w98:errorcluster)  [unwired: 10 in]
            n125 = Compound Arithmetic op=OR(w85, w89) -> (w90:bool)
            n126 = Select(t=string[] ["Exit"] ("f"), s=w90, f=string[] ["Run"] ("array")) -> (s? t:f=w100:string[])
            n127 = Build Array (concatenate)(w105, w100) -> (w103:string[])
          }
          frame "Exit" {
            # "Exit the Engine"
          }
        }
        n128 = Compound Arithmetic op=OR(w62, w64) -> (w63:bool)
      }
      frame Error {
      }
    }
  }
  n129 = Release Queue(queue=w22, error in (no error)=w23) -> (error out=w21:errorcluster)  [unwired: 1 in, 2 out]
  n130 = disable-structure shown="Disabled" {
    disable-tunnel: w24 -> [w491 _]
    disable-tunnel: w21 -> [w490 w492]
    disable-tunnel: [w489 w492] -> w20
    frame Disabled {
      n131 = call <vilib>:"TestStand - Close Termination Monitor.vi"("error in (no error)"=w490, "Status Monitor In"=w491) -> ("error out"=w489:errorcluster)  [unwired: 9 in]
    }
    frame Enabled {
    }
  }
  n132 = Close Reference(reference=w19, error in (no error)=w20) -> (error out=w14:errorcluster)
  n133 = call "Database Driver.vi"("Options"=w8, "error in"=w14) -> ("error out"=w10:errorcluster)  [unwired: 6 in, 3 out]
  n134 = call "Database Server Driver.vi"("Options"=w8, "error in"=w10) -> ("error out"=→"error out":errorcluster)  [unwired: 6 in, 3 out]
